vi "Tray Position計算.vi"(4 "¨ú®Æ¦ìPitch(Y¶b)":dbl, 5 "¨ú®Æ¦ìPitch(X¶b)":dbl, 6 "¨ú®Æ®Õ¥¿¦ì(Y¶b)":dbl, 7 "¨ú®Æ®Õ¥¿¦ì(X¶b)":dbl, 8 "error in (no error)":errorcluster, 10 "Col":i32, 11 "DataArray":bool[](array[boolean])) -> (0 "error out":errorcluster, 1 "DataArrayOut":bool[](array[boolean]), 2 "¨ú®Æ¦ì(Y¶b)":dbl, 3 "¨ú®Æ¦ì(X¶b)":dbl)   [LabVIEW 2015]
panel:
  out "¦C(X¶b)":i32
  out "¦æ(Y¶b)":i32
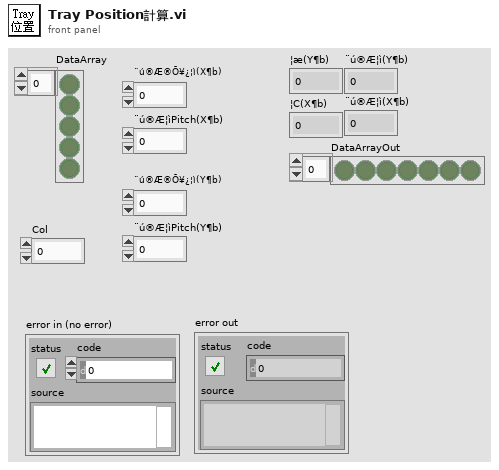
[diagram p1: front panel]
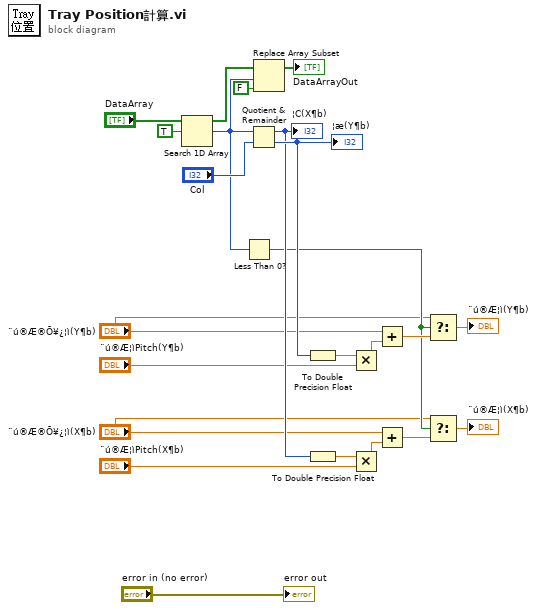
[diagram p0: block diagram]
diagram:
  n1 = Search 1D Array(1D array="DataArray", element=TRUE) -> (index of element=w8:i32)  [unwired: 1 in]
  n2 = Less Than 0?(x=w8) -> (x < 0?=w5:bool)
  n3 = Quotient & Remainder(x=w8, y="Col") -> (x-y*floor(x/y)=w15:i32, floor(x/y)=w20:i32)
  "¦æ(Y¶b)" <- w20
  "¦C(X¶b)" <- w15
  n4 = Replace Array Subset(array="DataArray", new element=FALSE ("new element/subarray"), index=w8) -> (→"DataArrayOut":bool[])
  n5 = To Double Precision Float(number=w20) -> (double precision float=w18:dbl)
  n6 = To Double Precision Float(number=w15) -> (double precision float=w17:dbl)
  n7 = Multiply(x=w18, y="¨ú®Æ¦ìPitch(Y¶b)") -> (x*y=w19:dbl)
  n8 = Multiply(x=w17, y="¨ú®Æ¦ìPitch(X¶b)") -> (x*y=w16:dbl)
  n9 = Add(x="¨ú®Æ®Õ¥¿¦ì(Y¶b)", y=w19) -> (x+y=w7:dbl)
  n10 = Add(x="¨ú®Æ®Õ¥¿¦ì(X¶b)", y=w16) -> (x+y=w4:dbl)
  n11 = Select(t="¨ú®Æ®Õ¥¿¦ì(Y¶b)", s=w5, f=w7) -> (s? t:f=→"¨ú®Æ¦ì(Y¶b)":dbl)
  n12 = Select(t="¨ú®Æ®Õ¥¿¦ì(X¶b)", s=w5, f=w4) -> (s? t:f=→"¨ú®Æ¦ì(X¶b)":dbl)
  "error out" <- "error in (no error)"
